vi "configure.vi"(8 "error in (no error)":errorcluster, 11 "ScanModeTS090821Circular2D in":refnum<class "ImagingModeTS090821Circular2D.lvclass">) -> (0 "error out":errorcluster, 3 "ScanModeTS090821Circular2D out":refnum<class "ImagingModeTS090821Circular2D.lvclass">)   [LabVIEW 2010, in "ImagingModeTS090821Circular2D.lvclass"]
doc: "The dynamic dispatch version of this VI loads and displays the configuration file associated with the plug-in object. The user modify and save the configuration data."
uses:
  ImagingModeTS090821Circular2D.lvclass
  ImagingModeDL090923Scaffold/ImagingModeDL090923Scaffold/component_configuration_visibility_cluster.ctl
  ImagingModeDL090923Scaffold/ImagingModeDL090923Scaffold/ImagingModeDL090923Scaffold.lvclass
  ImagingModeDL090923Scaffold/ImagingModeDL090923Scaffold/configuration_visibility_cluster.ctl
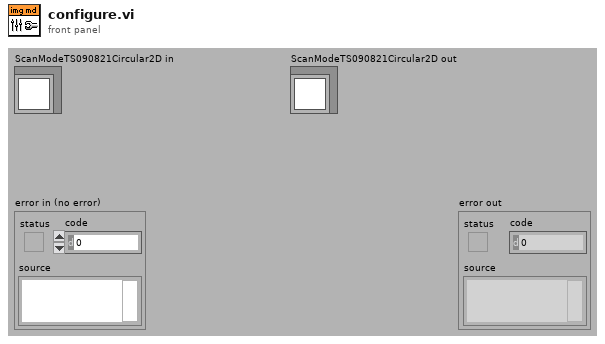
[diagram p1: front panel]
types:
  T1 = typedef "ImagingModeDL090923Scaffold.lvclass/configuration_visibility_cluster.ctl" = cluster{"Instrument":T2, "Trajectory":T2, "ScanHead":T2, "DAQ":T2, "ImageAssembler":T2, "DataCollection":T2, "Display":T2, "Analyser":T2, "Stimulator":T2, "enable Trajectory-to-ImageAssembler adapter":bool}
  T2 = typedef "ImagingModeDL090923Scaffold.lvclass/component_configuration_visibility_cluster.ctl" = cluster{"enable":bool, "enable adapter":bool}
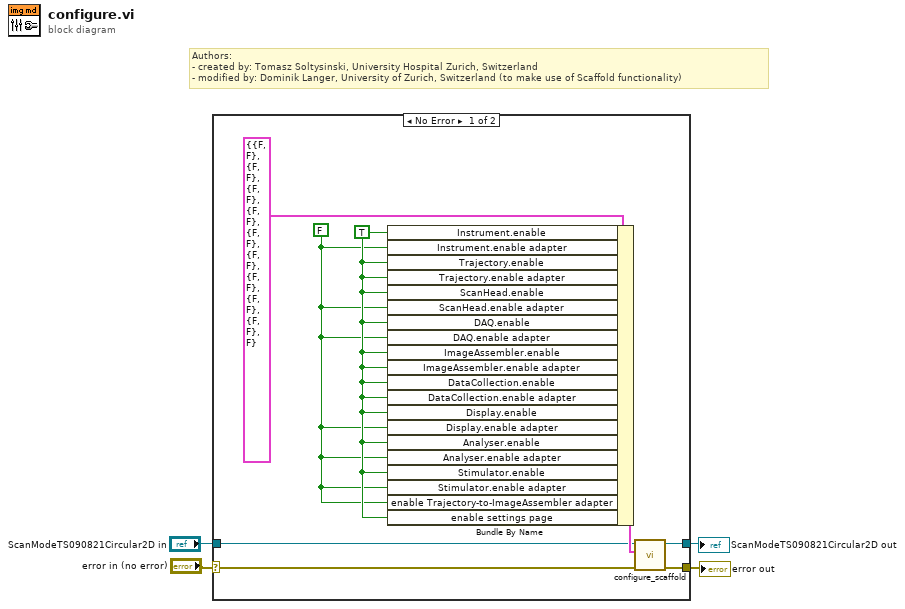
[diagram p0: block diagram]
diagram:
  # "Authors: \n- created by: Tomasz Soltysinski, University Hospital Zurich, Switzerland\n- modified by: Dominik Langer, University of Zurich, Switzerland (to make use of Scaffold functionality)"
  n1 = case shown="No Error" "error in (no error)" {
    selector: "error in (no error)" -> [w10 w14]
    tunnel: [w7 w14] -> w3
    tunnel: [w8 w13] -> w1
    tunnel: "ScanModeTS090821Circular2D in" -> [w9 w13]
    frame No Error {
      w5 = FALSE ("Instrument.enable adapter")
      w11 = TRUE ("Instrument.enable")
      n2 = Bundle By Name(cluster=T1 {"Instrument"={"enable"=FALSE, "enable adapter"=FALSE}, "Trajectory"={"enable"=FALSE, "enable adapter"=FALSE}, "ScanHead"={"enable"=FALSE, "enable adapter"=FALSE}, "DAQ"={"enable"=FALSE, "enable adapter"=FALSE}, "ImageAssembler"={"enable"=FALSE, "enable adapter"=FALSE}, "DataCollection"={"enable"=FALSE, "enable adapter"=FALSE}, "Display"={"enable"=FALSE, "enable adapter"=FALSE}, "Analyser"={"enable"=FALSE, "enable adapter"=FALSE}, "Stimulator"={"enable"=FALSE, "enable adapter"=FALSE}, "enable Trajectory-to-ImageAssembler adapter"=FALSE} ("visibilities"), "Instrument.enable"=w11, "Instrument.enable adapter"=w5, "Trajectory.enable"=w11, "Trajectory.enable adapter"=w11, "ScanHead.enable"=w11, "ScanHead.enable adapter"=w5, "DAQ.enable"=w11, "DAQ.enable adapter"=w5, "ImageAssembler.enable"=w11, "ImageAssembler.enable adapter"=w11, "DataCollection.enable"=w11, "DataCollection.enable adapter"=w11, "Display.enable"=w11, "Display.enable adapter"=w5, "Analyser.enable"=w11, "Analyser.enable adapter"=w5, "Stimulator.enable"=w11, "Stimulator.enable adapter"=w5, "enable Trajectory-to-ImageAssembler adapter"=w5, "enable settings page"=w11) -> (w12:T1)
      n3 = call-dynamic "configure_scaffold.vi"("error in (no error)"=w10, "visibilities"=w12, "ScanModeDL090923Scaffold in"=w9) -> ("error out"=w7:errorcluster, "ScanModeDL090923Scaffold out"=w8:refnum<class "ImagingModeTS090821Circular2D.lvclass">)  [unwired: 7 in]
    }
    frame Error {
    }
  }
  "error out" <- w3
  "ScanModeTS090821Circular2D out" <- w1
